vi "Write Browse Options Button Text.vi"(8 "error in (no error)":errorcluster, 10 "ButtonText":string, 11 "Path.lvclass in":refnum<class "Path.lvclass">) -> (0 "error out":errorcluster, 3 "Path.lvclass out":refnum<class "Path.lvclass">)   [LabVIEW 2015, in "Path.lvclass"]
uses:
  Path.lvclass
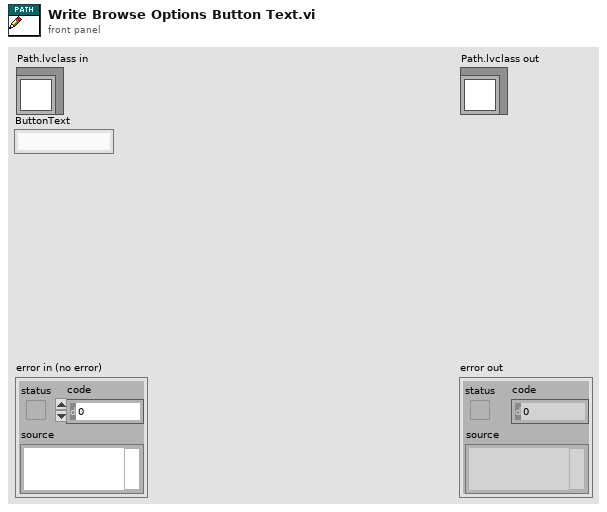
[diagram p1: front panel]
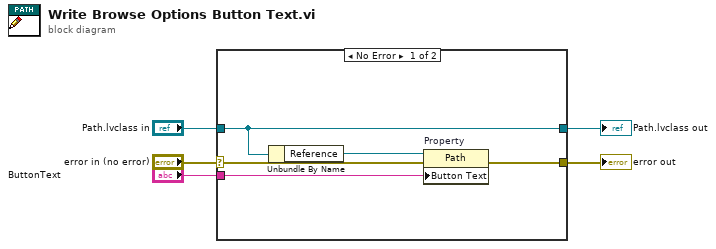
[diagram p0: block diagram]
diagram:
  n1 = case shown="No Error" "error in (no error)" {
    selector: "error in (no error)" -> [w6 w12]
    tunnel: [w10 w12] -> w4
    tunnel: [w8 w11] -> w2
    tunnel: "Path.lvclass in" -> [w8 w11]
    tunnel: "ButtonText" -> [w9 _]
    frame No Error {
      n2 = Unbundle By Name(w8) -> ("Reference"=w7:refnum<vi>)
      n3 = property on="Property" class="Path"(reference=w7, error in=w6, "Button Text"=w9) -> (error out=w10:errorcluster)  [unwired: 1 out]
    }
    frame Error {
    }
  }
  "error out" <- w4
  "Path.lvclass out" <- w2
